vi "Create Random Data.vi"(1 "Number of rounds":dbl=21.0) -> (0 "Output [tag_id, anchor_id, distance, time]":dbl[][](array[numeric]))   [LabVIEW 2014]
uses:
  Anchor/Anchor.lvclass
panel:
  out "anchor id":dbl
  out "y":dbl[](array[numeric])
  out "x":dbl[](array[numeric])
  out "Array":dbl[][](array[numeric])
  out "Array 2":cluster{"x":dbl, "y":dbl, "v":dbl, "h":dbl}[](array[cluster])
  out "A2 id":dbl
  out "A3 id":dbl
  out "A1 id":dbl
  out "A2 y":dbl
  out "A2 x":dbl
  out "A3 y":dbl
  out "A3 x":dbl
  out "A1 y":dbl
  out "A1 x":dbl
  in  "Path":path=path "C:/Users/Marvin/Documents/SPLAT/smooth_data.txt"
  out "error out":errorcluster
  in  "error in":errorcluster
  out "Subtracted time id2":dbl
  out "Subtracted time id0":dbl
  out "Subtracted time id1":dbl
  out "sample time":timestamp
  out "Distance":dbl
  out "Distance 2":dbl
  out "Y end randomized":dbl
  out "X end randomized":dbl
  out "Distance":dbl
  out "anchor id":dbl
  in  "Anchor 2":refnum<class "Anchor.lvclass">=refnum caption="The result is a created anchor"
  in  "Anchor 3":refnum<class "Anchor.lvclass">=refnum caption="The result is a created anchor"
  in  "Anchor 1":refnum<class "Anchor.lvclass">=refnum caption="The result is a created anchor"
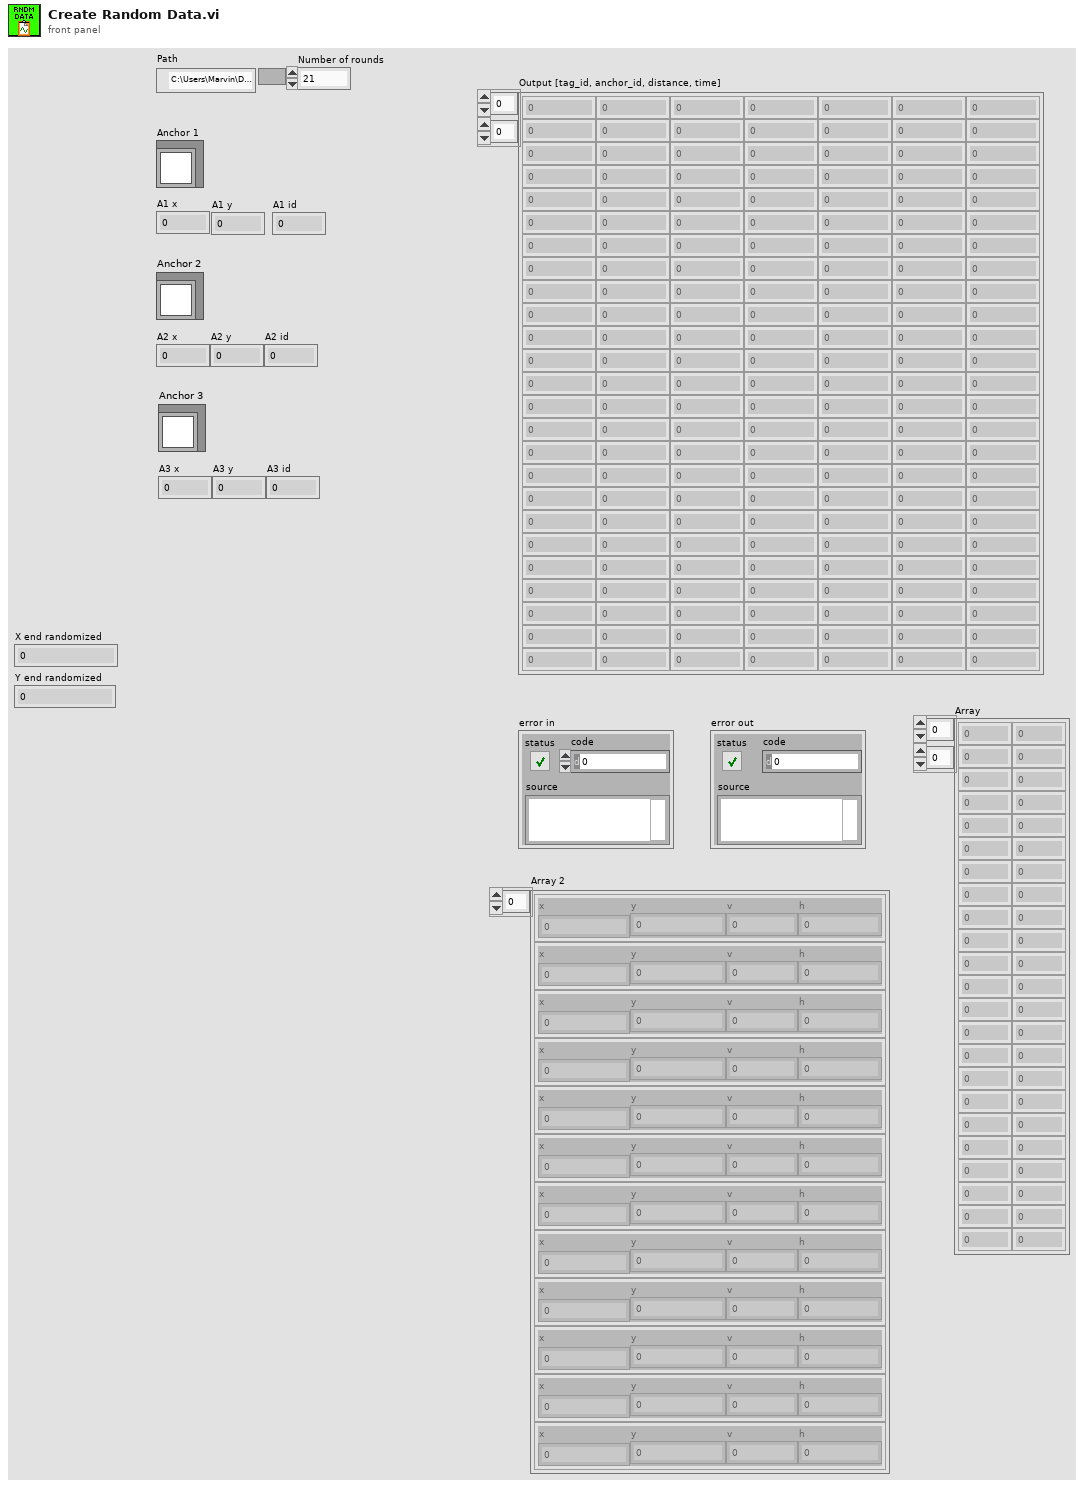
[diagram p1: front panel]
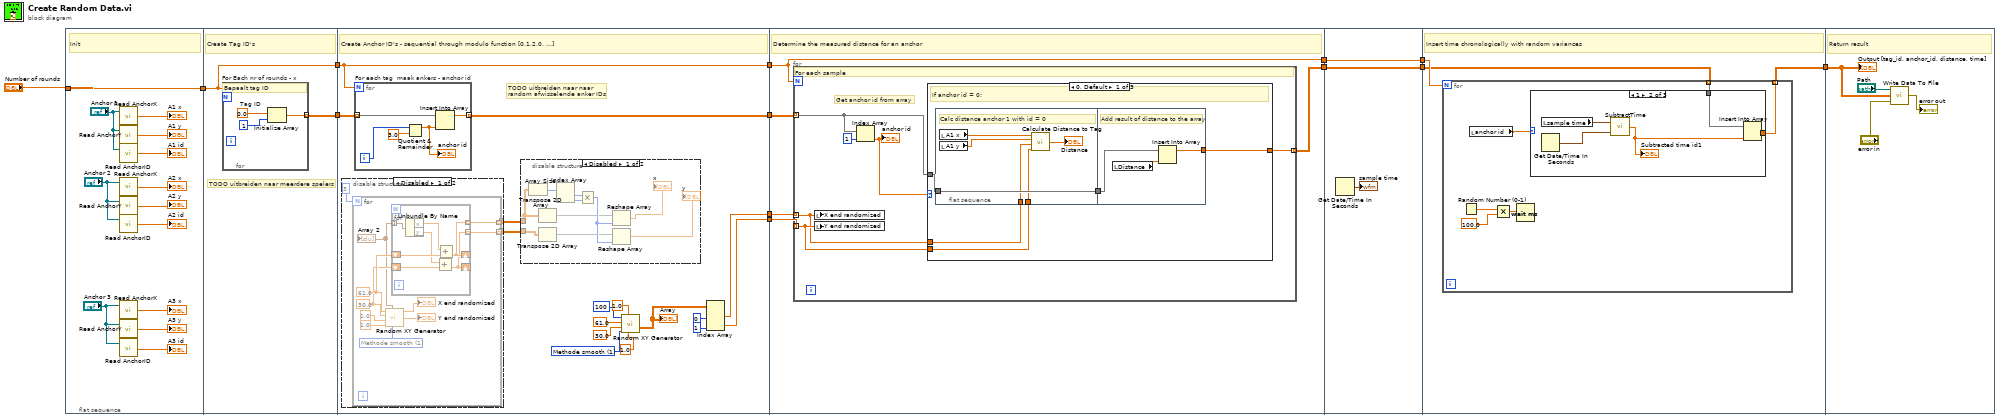
[diagram p0: block diagram]
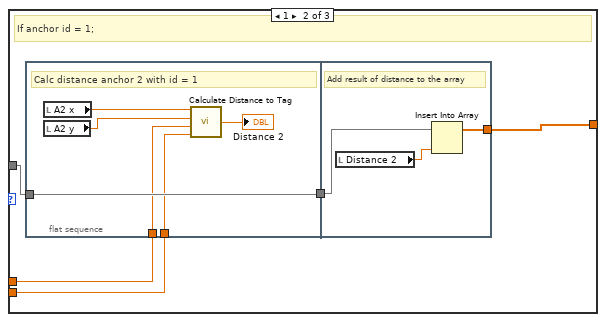
[diagram p4: hidden frame]
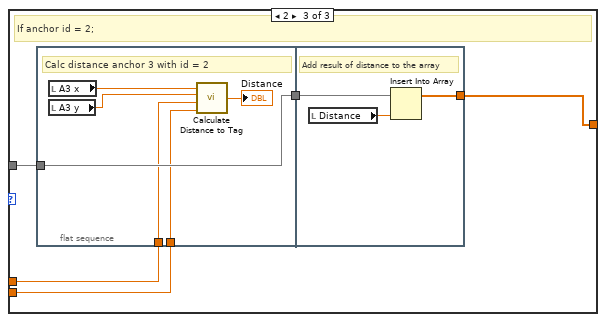
[diagram p5: hidden frame]
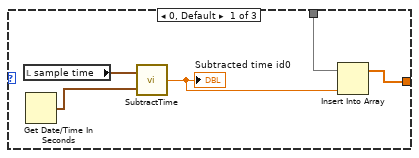
[diagram p6: hidden frame]
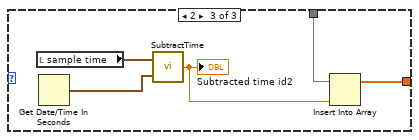
[diagram p7: hidden frame]
diagram:
  n1 = flat-sequence {
    tunnel: "Number of rounds" -> [w26]
    tunnel: [w26] -> w13
    tunnel: [w28] -> w12
    tunnel: [w27] -> w11
    tunnel: w13 -> [w27]
    tunnel: w12 -> [w47]
    tunnel: [w46] -> w10
    tunnel: w11 -> [w45]
    tunnel: [w45] -> w9
    tunnel: [w38] -> w8
    tunnel: [w37] -> w7
    tunnel: w10 -> [w87]
    tunnel: w9 -> [w85]
    tunnel: [w86] -> w6
    tunnel: [w85] -> w5
    tunnel: w8 -> [w84]
    tunnel: w7 -> [w83]
    tunnel: w6 -> [w138]
    tunnel: [w138] -> w4
    tunnel: w5 -> [w137]
    tunnel: [w137] -> w3
    tunnel: w4 -> [w140]
    tunnel: w3 -> [w141]
    tunnel: [w139] -> w2
    tunnel: w2 -> [w163]
    frame #0 {
      # "Init"
      n2 = call-dynamic "Read AnchorX.vi"("Anchor in"="Anchor 1") -> ("AnchorX"=→"A1 x":dbl)  [unwired: 1 in, 2 out]
      n3 = call-dynamic "Read AnchorY.vi"("Anchor in"="Anchor 1") -> ("AnchorY"=→"A1 y":dbl)  [unwired: 1 in, 2 out]
      n4 = call-dynamic "Read AnchorID.vi"("Anchor in"="Anchor 1") -> ("AnchorID"=→"A1 id":dbl)  [unwired: 1 in, 2 out]
      n5 = call-dynamic "Read AnchorX.vi"("Anchor in"="Anchor 2") -> ("AnchorX"=→"A2 x":dbl)  [unwired: 1 in, 2 out]
      n6 = call-dynamic "Read AnchorY.vi"("Anchor in"="Anchor 2") -> ("AnchorY"=→"A2 y":dbl)  [unwired: 1 in, 2 out]
      n7 = call-dynamic "Read AnchorID.vi"("Anchor in"="Anchor 2") -> ("AnchorID"=→"A2 id":dbl)  [unwired: 1 in, 2 out]
      n8 = call-dynamic "Read AnchorX.vi"("Anchor in"="Anchor 3") -> ("AnchorX"=→"A3 x":dbl)  [unwired: 1 in, 2 out]
      n9 = call-dynamic "Read AnchorY.vi"("Anchor in"="Anchor 3") -> ("AnchorY"=→"A3 y":dbl)  [unwired: 1 in, 2 out]
      n10 = call-dynamic "Read AnchorID.vi"("Anchor in"="Anchor 3") -> ("AnchorID"=→"A3 id":dbl)  [unwired: 1 in, 2 out]
    }
    frame #1 {
      # "TODO uitbreiden naar meerdere spelers"
      # "Create Tag ID's"
      n11 = for "For Each nr of rounds - x" {
        N: w27 -> [_]
        tunnel: [w30] -> w28 mode=indexing
        w31 = 0.0  # Tag ID
        # "Bepaalt tag ID"
        n12 = Initialize Array ("Initialize Tag ID Row Array")(w31, 1 ("dimension size")) -> (w30:dbl[])
      }
    }
    frame #2 {
      w42 = u16 1 items=["Methode Random", "Methode smooth"] ("Random Methode")
      # "TODO uitbreiden naar naar \nrandom afwisselende anker IDs"
      # "Create Anchor ID's - sequential through modulo function [0,1,2,0, ...]"
      n13 = disable-structure shown="Disabled" {
        disable-tunnel: [w59 _] -> w44
        disable-tunnel: [w58 _] -> w43
        frame Disabled {
          n14 = for {
            N: 3 -> [_]
            tunnel: [w68] -> w59 mode=indexing
            tunnel: [w67] -> w58 mode=indexing
            w64 = u16 1 items=["Methode Random", "Methode smooth"] ("Random Methode")
            w62 = 30.0 ("Y start")
            w63 = 61.0 ("X start")
            n15 = call "Random XY Generator.vi"("X start"=w63, "Random Methode"=w64, "Y start"=w62, "Max V variatie"=1.0, "Max h variatie"=1.0) -> ("Array"=w61:cluster{"x":dbl, "y":dbl, "v":dbl, "h":dbl}[], "X end randomized"=→"X end randomized":dbl, "Y end randomized"=→"Y end randomized":dbl)  [unwired: 1 out]
            "Array 2" <- w61
            n16 = for {
              tunnel: w61 -> [w77] mode=indexing
              tunnel: [w73] -> w67 mode=indexing
              tunnel: [w71] -> w68 mode=indexing
              shift-right: [w73] -> _
              shift-left: w63 -> [w76]
              shift-right: [w71] -> _
              shift-left: w62 -> [w75]
              n17 = Unbundle By Name(w77) -> ("x"=w74:dbl, "y"=w72:dbl)
              n18 = Add(x=w72, y=w75) -> (x+y=w71:dbl)
              n19 = Add(x=w74, y=w76) -> (x+y=w73:dbl)
            }
          }
        }
        frame Enabled {
        }
      }
      n20 = for "For each tag  maak ankers - anchor id" {
        N: w45 -> [_]
        tunnel: w47 -> [w82] mode=indexing
        tunnel: [w81] -> w46 mode=indexing
        i -> [w79]
        n21 = Quotient & Remainder(x=w79, y=3.0 ("x")) -> (x-y*floor(x/y)=w78:dbl)  [unwired: 1 out]
        "anchor id" <- w78
        n22 = Insert Into Array(array=w82, new element=w78) -> (w81:dbl[])  [unwired: 1 in]
      }
      n23 = disable-structure shown="Disabled" {
        disable-tunnel: w44 -> [w49 _]
        disable-tunnel: w43 -> [w48 _]
        frame Disabled {
          n24 = Array Size(array=w48) -> (size(s)=w55:i32[])
          n25 = Transpose 2D Array(2D array=w48) -> (transposed array=w50:dbl[][])
          n26 = Transpose 2D Array(2D array=w49) -> (transposed array=w51:dbl[][])
          n27 = Index Array(array=w55) -> (element #1=w54:i32, element #2=w53:i32)  [unwired: 2 in]
          n28 = Multiply(x=w54, y=w53) -> (x*y=w52:i32)
          n29 = Reshape Array(w51, w52) -> (→"y":dbl[])
          n30 = Reshape Array(w50, w52) -> (→"x":dbl[])
        }
        frame Enabled {
        }
      }
      n31 = call "Random XY Generator.vi"("Max h variatie"=1.0 ("Max V variatie"), "Max V variatie"=1.0 ("Max h variatie"), "Random Methode"=w42, "Y start"=30.0, "X start"=61.0, "number of rounds"=100) -> ("Array"=w41:dbl[][])  [unwired: 3 out]
      "Array" <- w41
      n32 = Index Array(array=w41, index (col) #1=0 ("disabled index (col)"), index (col) #2=1 ("index (col)")) -> (element #1=w38:dbl[], element #2=w37:dbl[])  [unwired: 2 in]
    }
    frame #3 {
      # "Determine the measured distance for an anchor"
      n33 = for {
        N: w85 -> [_]
        tunnel: w87 -> [w92] mode=indexing
        tunnel: [w93] -> w86 mode=indexing
        tunnel: w84 -> [w88] mode=indexing
        tunnel: w83 -> [w89] mode=indexing
        # "Get anchor id from array"
        # "For each sample"
        n34 = local write "X end randomized"(w88) -> ()
        n35 = local write "Y end randomized"(w89) -> ()
        n36 = Index Array(array=w92, index=1) -> (element=w90:dbl)
        "anchor id" <- w90
        n37 = case shown="0, Default" w90 {
          tunnel: w92 -> [w98 w111 w125]
          tunnel: [w96 w110 w124] -> w93
          tunnel: w89 -> [w95 w108 w122]
          tunnel: w88 -> [w94 w109 w123]
          frame 0, Default {
            # "If anchor id = 0;"
            n38 = flat-sequence {
              tunnel: w98 -> [w104]
              tunnel: [w104] -> w97
              tunnel: w95 -> [w100]
              tunnel: w94 -> [w99]
              tunnel: w97 -> [w107]
              tunnel: [w105] -> w96
              frame #0 {
                # "Calc distance anchor 1 with id = 0"
                n39 = local read "A1 x"() -> (w103:dbl)
                n40 = local read "A1 y"() -> (w102:dbl)
                n41 = call "Calculate Distance to Tag.vi"("Tag y"=w100, "Tag x"=w99, "Anchor y"=w102, "Anchor x"=w103) -> ("Distance"=→"Distance":dbl)
              }
              frame #1 {
                # "Add result of distance to the array"
                n42 = local read "Distance"() -> (w106:dbl)
                n43 = Insert Into Array(array=w107, new element=w106) -> (w105:dbl[])  [unwired: 1 in]
              }
            }
          }
          frame 1 {
            # "If anchor id = 1;"
            n44 = flat-sequence {
              tunnel: [w118] -> w112
              tunnel: w111 -> [w118]
              tunnel: w109 -> [w114]
              tunnel: w108 -> [w113]
              tunnel: w112 -> [w121]
              tunnel: [w119] -> w110
              frame #0 {
                # "Calc distance anchor 2 with id = 1"
                n45 = local read "A2 x"() -> (w117:dbl)
                n46 = local read "A2 y"() -> (w116:dbl)
                n47 = call "Calculate Distance to Tag.vi"("Tag y"=w113, "Tag x"=w114, "Anchor y"=w116, "Anchor x"=w117) -> ("Distance"=→"Distance 2":dbl)
              }
              frame #1 {
                # "Add result of distance to the array"
                n48 = local read "Distance 2"() -> (w120:dbl)
                n49 = Insert Into Array(array=w121, new element=w120) -> (w119:dbl[])  [unwired: 1 in]
              }
            }
          }
          frame 2 {
            # "If anchor id = 2;"
            n50 = flat-sequence {
              tunnel: [w132] -> w126
              tunnel: w125 -> [w132]
              tunnel: w123 -> [w128]
              tunnel: w122 -> [w127]
              tunnel: w126 -> [w135]
              tunnel: [w133] -> w124
              frame #0 {
                # "Calc distance anchor 3 with id = 2"
                n51 = local read "A3 x"() -> (w131:dbl)
                n52 = local read "A3 y"() -> (w130:dbl)
                n53 = call "Calculate Distance to Tag.vi"("Tag y"=w127, "Tag x"=w128, "Anchor y"=w130, "Anchor x"=w131) -> ("Distance"=→"Distance":dbl)
              }
              frame #1 {
                # "Add result of distance to the array"
                n54 = local read "Distance"() -> (w134:dbl)
                n55 = Insert Into Array(array=w135, new element=w134) -> (w133:dbl[])  [unwired: 1 in]
              }
            }
          }
        }
      }
    }
    frame #4 {
      n56 = Get Date/Time In Seconds() -> (seconds since 1Jan1904=→"sample time":timestamp)
    }
    frame #5 {
      # "Insert time chronologically with random variances"
      n57 = for {
        N: w141 -> [_]
        tunnel: w140 -> [w146] mode=indexing
        tunnel: [w145] -> w139 mode=indexing
        n58 = Random Number (0-1)() -> (number: 0 to 1=w143:dbl)
        n59 = local read "anchor id"() -> (w147:dbl)
        n60 = Multiply(x=w143, y=100.0) -> (x*y=w142:dbl)
        n61 = Wait (ms)(milliseconds to wait=w142) -> ()  [unwired: 1 out]
        n62 = case shown="1" w147 {
          tunnel: w146 -> [w150 w157 w160]
          tunnel: [w148 w155 w158] -> w145
          frame 0, Default {
            n63 = local read "sample time"() -> (w152:timestamp)
            n64 = Get Date/Time In Seconds() -> (seconds since 1Jan1904=w151:timestamp)
            n65 = call "SubtractTime.vi"("New Time Stamp"=w151, "Old Time Stamp"=w152) -> ("Subtracted time"=w149:dbl)
            "Subtracted time id0" <- w149
            n66 = Insert Into Array(array=w150, new element=w149) -> (w148:dbl[])  [unwired: 1 in]
          }
          frame 1 {
            n67 = local read "sample time"() -> (w153:timestamp)
            n68 = Get Date/Time In Seconds() -> (seconds since 1Jan1904=w154:timestamp)
            n69 = call "SubtractTime.vi"("New Time Stamp"=w154, "Old Time Stamp"=w153) -> ("Subtracted time"=w156:dbl)
            "Subtracted time id1" <- w156
            n70 = Insert Into Array(array=w157, new element=w156) -> (w155:dbl[])  [unwired: 1 in]
          }
          frame 2 {
            n71 = local read "sample time"() -> (w162:timestamp)
            n72 = Get Date/Time In Seconds() -> (seconds since 1Jan1904=w161:timestamp)
            n73 = call "SubtractTime.vi"("New Time Stamp"=w161, "Old Time Stamp"=w162) -> ("Subtracted time"=w159:dbl)
            "Subtracted time id2" <- w159
            n74 = Insert Into Array(array=w160, new element=w159) -> (w158:dbl[])  [unwired: 1 in]
          }
        }
      }
    }
    frame #6 {
      # "Return result"
      n75 = call "Write Data To File.vi"("error in"="error in", "Array"=w163, "file path (use dialog)"="Path") -> ("error out"=→"error out":errorcluster)
      "Output [tag_id, anchor_id, distance, time]" <- w163
    }
  }
